vi "Read Root Lifetime.vi"(11 "Actor in":refnum<class "Actor.lvclass">) -> (2 "Root Lifetime":T1)   [LabVIEW 2025]
uses:
  Actor.lvclass
  Root Lifetime.ctl
  jettl.lvlib
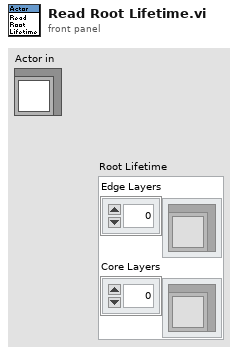
[diagram p1: front panel]
types:
  T1 = typedef "jettl.lvlib/Root Lifetime.ctl" = cluster{"Edge Layers":refnum<class "Actor.lvclass">[], "Core Layers":refnum<class "Actor.lvclass">[]}
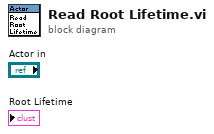
[diagram p0: block diagram]
diagram:
